vi "Put Time Alarm V.vi"(8 "error in (no error)":errorcluster, 11 "timeAlarm":string) -> (0 "error out":errorcluster, 2 "function return":i16, 3 "timeAlarm out":string)   [LabVIEW 2009, in "VantagePro.lvlib"]
doc: "DllAccess short int _stdcall PutTimeAlarm_V (char* timeAlarm);"
uses:
  VantagePro.lvlib
  <userlib>/VantagePro/VantagePro.dll
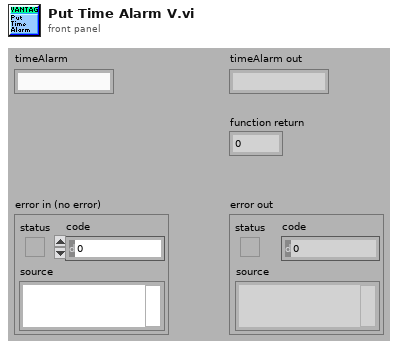
[diagram p1: front panel]
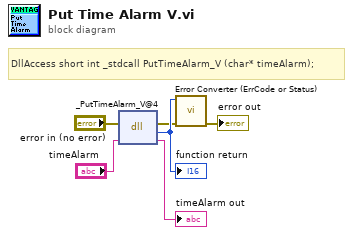
[diagram p0: block diagram]
diagram:
  # "DllAccess short int _stdcall PutTimeAlarm_V (char* timeAlarm);"
  n1 = dll-call lib="C:/Program Files/National Instruments/LabVIEW 2010/user.lib/VantagePro/VantagePro.*" fn="_PutTimeAlarm_V@4"(error in="error in (no error)", "timeAlarm"="timeAlarm") -> (error out=w2:errorcluster, w6:i16, "timeAlarm"=→"timeAlarm out":string)  [unwired: 2 in, 1 out]
  "function return" <- w6
  n2 = call "Error Converter (ErrCode or Status).vi"("error in (no error)"=w2, "error code"=w6) -> ("error out"=→"error out":errorcluster)  [unwired: 9 in]
